vi "acquisition_typedef.vi"(8 "error in":errorcluster, 11 "command":string) -> (0 "error out":errorcluster, 3 "data value reference":refnum<data-value>)   [LabVIEW 2010]
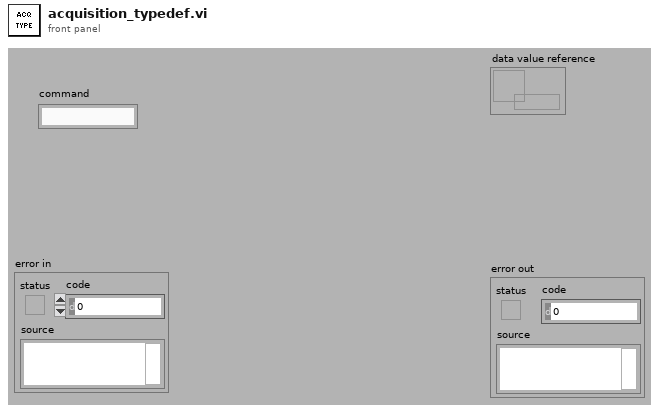
[diagram p1: front panel]
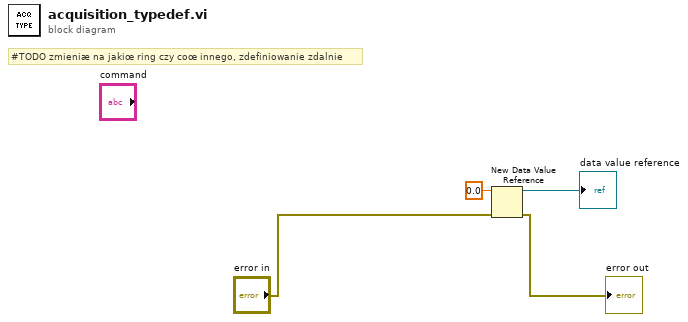
[diagram p0: block diagram]
diagram:
  # "#TODO zmieniæ na jakiœ ring czy coœ innego, zdefiniowanie zdalnie"
  n1 = New Data Value Reference(data value=0.0, error in="error in") -> (data value reference=→"data value reference":refnum<data-value>, error out=→"error out":errorcluster)
